vi "Set Sensitivity (High BW I Mode).vi"(8 "error in (no error)":errorcluster, 10 "Sensitivity IMODE1":T1=enum."5 fA", 11 "VISA resource name":refnum<visa-resource-name>) -> (0 "error out":errorcluster, 3 "VISA resource name out":refnum<visa-resource-name>)   [LabVIEW 2019, in "SR7270 Drivers.lvlib"]
uses:
  SR7270 Drivers.lvlib
  Typedefs/SEN-IMODE1--enum.ctl
  Typedefs/IMODE--enum.ctl
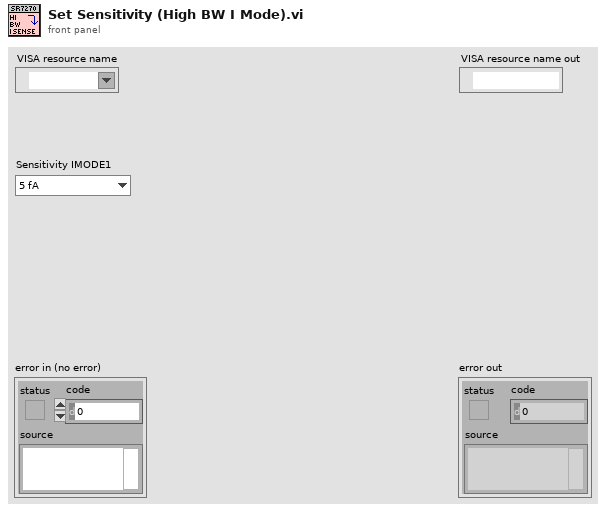
[diagram p1: front panel]
types:
  T1 = typedef "SR7270 Drivers.lvlib/SEN-IMODE1--enum.ctl" = enum16{"2 fA", "5 fA", "10 fA", "20 fA", "50 fA", "100 fA", "200 fA", "500 fA", "1 pA", "2 pA", "5 pA", "10 pA", "20 pA", "50 pA", "100 pA", "200 pA", "500 pA", "1 nA", "2 nA", "5 nA", "10 nA", "20 nA", "50 nA", "100 nA", "200 nA", "500 nA", "1 µA"}
  T2 = typedef "SR7270 Drivers.lvlib/IMODE--enum.ctl" = enum16{"Current Mode Off", "High bandwidth current mode", "Low noise current mode"}
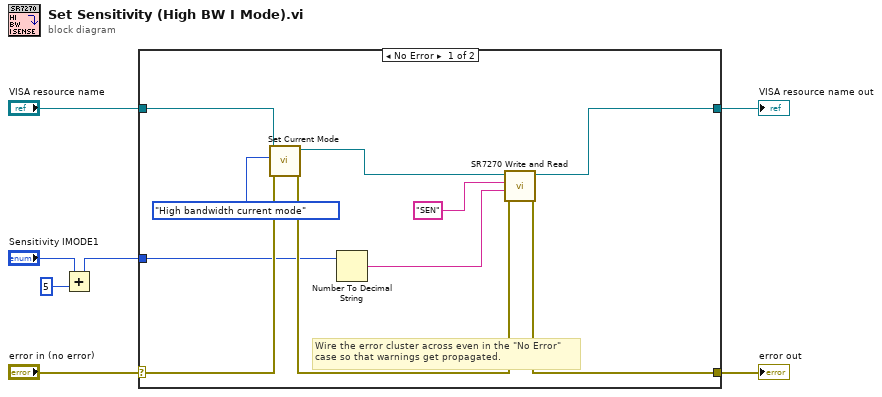
[diagram p0: block diagram]
diagram:
  n1 = Add(x="Sensitivity IMODE1", y=5) -> (x+y=w1:i32)
  n2 = case shown="No Error" "error in (no error)" {
    selector: "error in (no error)" -> [w15 w19]
    tunnel: [w13 w19] -> w7
    tunnel: [w8 w18] -> w6
    tunnel: "VISA resource name" -> [w10 w18]
    tunnel: w1 -> [w12 _]
    frame No Error {
      # "Wire the error cluster across even in the \"No Error\"\ncase so that warnings get propagated."
      n3 = call "Set Current Mode.vi"("error in (no error)"=w15, "Current Mode"=IMODE--enum."High bandwidth current mode", "VISA resource name"=w10) -> ("error out"=w14:errorcluster, "VISA resource name out"=w9:refnum<visa-resource-name>)  [unwired: 7 in]
      n4 = Number To Decimal String(number=w12) -> (decimal integer string=w11:string)  [unwired: 1 in]
      n5 = call "SR7270 Write and Read.vi"("error in (no error)"=w14, "Parameter(s)"=w11, "Command Name"="SEN", "VISA resource name"=w9) -> ("error out"=w13:errorcluster, "VISA resource name out"=w8:refnum<visa-resource-name>)  [unwired: 4 in, 2 out]
    }
    frame Error {
    }
  }
  "error out" <- w7
  "VISA resource name out" <- w6
